vi "UCL.vi"(0 "System no.":i32=1 min=1 max=4 step=1, 2 "Command Level":T1, 3 "Password":string, 5 "error in":errorcluster) -> (19 "error out":errorcluster)   [LabVIEW 2020]
doc: "UCL (Set User Command Level)\n\nDescription\nChanges the active user command level for the GCS interpreter of the communication interface \nused.\nThe active user command level of the GCS interpreter determines which commands are \navailable on the interface and for which parameters read and write access is granted.\n\nFormat\nUCL <User Command Level>[ <Password>]\n\nArguments\n<User Command Level>\nA user command level of the GCS interpreter\nThe available user command levels can be queried with USG? PROP (p. 79). The response lists \nthe user command levels according to the scope of the permissions associated with them. The \nscope of the permissions increases from top to bottom. A level includes the permissions of all \nlevels above it. \nPossible values: USR, ADV, FAY, DEV\nSee the table below for more details\n<Password>\nThe password required to change to the corresponding user command level\nPossible values: See table\nPermissions and passwords for the individual user command levels:\nUser command level Permissions Password\nUSR User Level\nAccessible are functionalities for normal operation \nand settings that must be adjustable in normal \noperation (e.g. parameters for adjusting the control \ncharacteristics).\nNo password \nrequired\nADV Expert Customer\nAccessible are the functionalities and settings of the \nlevel USR as well as all parameters and commands \nthe user needs for the configuration\nADVANCED\nFAY Only PI Staff\nPI-internal use\n-\nDEV Only FW Developers\nPI-internal use\n-\n\nResponse\nnone\n\nNotes\nThe UCL? command (p. 71) queries the active user command level for the GCS interpreter of the \ncommunication interface used.\nUsing the USG? PAM (p. 77) command, the available parameters (p. 119) and their properties \ncan be queried. The response includes, among other things, the user command level for the \nread access (<READ-UCL> column) and write access (<WRITE-UCL> column) to the parameter.\n\nUser command level\nUSR"
uses:
  UserCommandLevel.ctl
panel:
  # "UCL (Set User Command Level)\n\nChanges the active user command level for the GCS interpreter of the communication interface used.\nThe active user command level of the GCS interpreter determines which commands are available on the interface and for which parameters read and write access is granted."
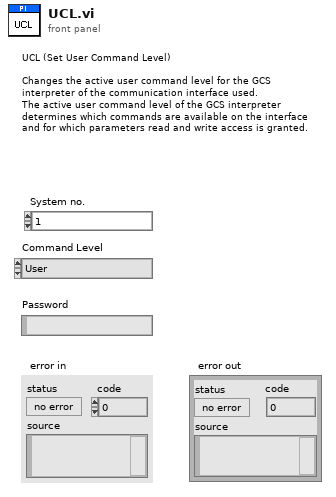
[diagram p1: front panel]
types:
  T1 = typedef "UserCommandLevel.ctl" = enum16{"User", "Expert", "PI Staff", "FW Developer"}
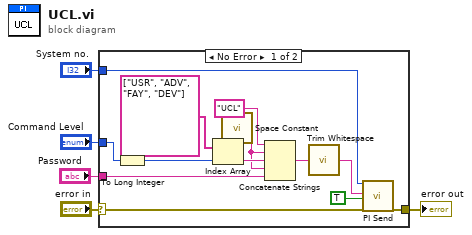
[diagram p0: block diagram]
diagram:
  n1 = case shown="No Error" "error in" {
    selector: "error in" -> [w18 w19]
    tunnel: [w15 w19] -> w5
    tunnel: "System no." -> [w17 _]
    tunnel: "Command Level" -> [w7 _]
    tunnel: "Password" -> [w9 _]
    frame No Error {
      n2 = To Long Integer(number=w7) -> (32bit integer=w6:i32)
      n3 = Index Array(array=string[] ["USR", "ADV", "FAY", "DEV"], index=w6) -> (element=w11:string)
      n4 = call "Space Constant.vi"() -> ("String"=w10:string)
      n5 = Concatenate Strings("UCL", w10, w11, w10, w9) -> (w13:string)
      n6 = call "Trim Whitespace.vi"("string"=w13) -> ("trimmed string"=w8:string)  [unwired: 1 in]
      n7 = call "PI Send.vi"("System no."=w17, "String to send"=w8, "Attach termination char.?"=TRUE, "error in"=w18) -> ("error out"=w15:errorcluster)  [unwired: 14 in, 1 out]
    }
    frame Error {
    }
  }
  "error out" <- w5
